vi "Read in last_sessionXML.vi"(8 "error in":errorcluster) -> (0 "error out":errorcluster, 3 "All Controlls For Saving":T1={"Confocal Controls"={"Channel Selection"=enum."A", "Pixel Count"={"Pixels in X"=512, "Pixels in Y"=512}, "Field Size"=174.0, "Frames"=0, "Averaging"=FALSE, "Alignment"=0.0, "Scan Mode"=TRUE, "Gain"={"Gain A"=0, "Gain B"=0}, "Enable PMTs"={"A"=TRUE, "B"=TRUE}, "Voltage Range"={"Range A"=10, "Range B"=10}, "Multi Frame Count"=0.0, "Trigger Mode"=2.0, "Real Time Averaging"=TRUE, "PFOV"=0.0, "MicronsPerPx"=0.0}, "iFlex Control"={"561"=0.0, "488"=0.0, "Global Shutter"=FALSE, "561 Shutter"=FALSE}, "PIFOC Settings"={"PIFOC Position (mm) [SET]"=0.0, "PIFOC Position\n(um) [ACT]"=0.0087, "last command"=""}, "PinSelector"=6.0, "Manlight Controls"={"Manlight Power"=0.0, "Open Serial"=FALSE, "VISA Refnum"=""}, "Exp Params"={"Experiment Type"="2D Snapshot", "Experiment Name"="Experiment_1", "ExpPath"=path "E:/Data", "TSFrames"=1000, "TSfps"=1000, "ZTSFrames"=1000, "ZTSdt"=1, "Streaming"=FALSE, "Z Stack Settings"={"Start"=0.0, "Step Size"=0.1, "Finish"=1.0}, "total images"=1, "tdms ref"=refnum, "frame #"=0, "images per stack"=1, "total stacks"=1, "period"=1, "PI MVR Increment"=""}, "Spots"=[]} {"Spots"."Z" format="%_4g"; "Spots"."Y" format="%_4g"; "Spots"."X" format="%_4g"; "Spots"."Phase" format="%_4g"; "Spots"."Intensity" format="%_4g"; "Exp Params"."period" min=1; "Exp Params"."total stacks" min=1; "Exp Params"."images per stack" min=1; "Exp Params"."total images" min=1; "Exp Params"."Z Stack Settings"."Start" min=0.0 max=100.0 step=0.1; "Exp Params"."Z Stack Settings"."Step Size" min=0.1 max=100.0 step=0.1; "Exp Params"."Z Stack Settings"."Finish" min=0.0 max=100.0 step=0.1; "Exp Params"."TSFrames" min=1 step=1; "Exp Params"."ZTSdt" min=1 step=1; "Exp Params"."ZTSFrames" min=2 step=1; "Exp Params"."TSfps" min=1 max=1000 step=1; "Manlight Controls"."Manlight Power" min=0.0 max=10.0 step=0.1 scale=0.0..10.0; "PinSelector" items=["25", "30", "35", "40", "45", "50", "60", "70", "80", "90", "100", "125", "200", "300", "1000", "2000"]; "PIFOC Settings"."PIFOC Position\n(um) [ACT]" format="%.2f"; "PIFOC Settings"."PIFOC Position (mm) [SET]" min=0.0 max=100.0 step=0.1 scale=0.0..100.0; "iFlex Control"."561" min=12.5 max=100.0 step=0.1 scale=0.0..100.0; "iFlex Control"."488" min=30.0 max=100.0 step=0.1 scale=0.0..100.0; "Confocal Controls"."Field Size" min=5.0 max=255.0 step=1.0 scale=5.0..255.0; "Confocal Controls"."PFOV" min=1.0 max=300.0 step=0.1; "Confocal Controls"."MicronsPerPx" min=0.01 step=0.01 format="%.2f"; "Confocal Controls"."Gain"."Gain B" min=1 max=100 step=1; "Confocal Controls"."Gain"."Gain A" min=1 max=100 step=1; "Confocal Controls"."Voltage Range"."Range B" items=["100mV"=5, "200mV"=6, "400mV"=7, "1V"=10, "2V"=11, "4V"=12]; "Confocal Controls"."Voltage Range"."Range A" items=["100mV"=5, "200mV"=6, "400mV"=7, "1V"=10, "2V"=11, "4V"=12]; "Confocal Controls"."Pixel Count"."Pixels in Y" items=["32"=32, "64"=64, "128"=128, "256"=256, "512"=512, "1024"=1024, "2048"=2048]; "Confocal Controls"."Pixel Count"."Pixels in X" items=["32"=32, "64"=64, "128"=128, "256"=256, "512"=512, "1024"=1024, "2048"=2048]})   [LabVIEW 2020]
uses:
  _Controls/All Controls For Saving.ctl
  _Controls/Confocal Controls.ctl
  _Controls/iFlex.ctl
  _Controls/PIFOC Position.ctl
  _Controls/Manlight Controls.ctl
  _Controls/Exp Params.ctl
  _Controls/Spots.ctl
  <vilib>/Utility/xml.llb/Read From XML File(string).vi
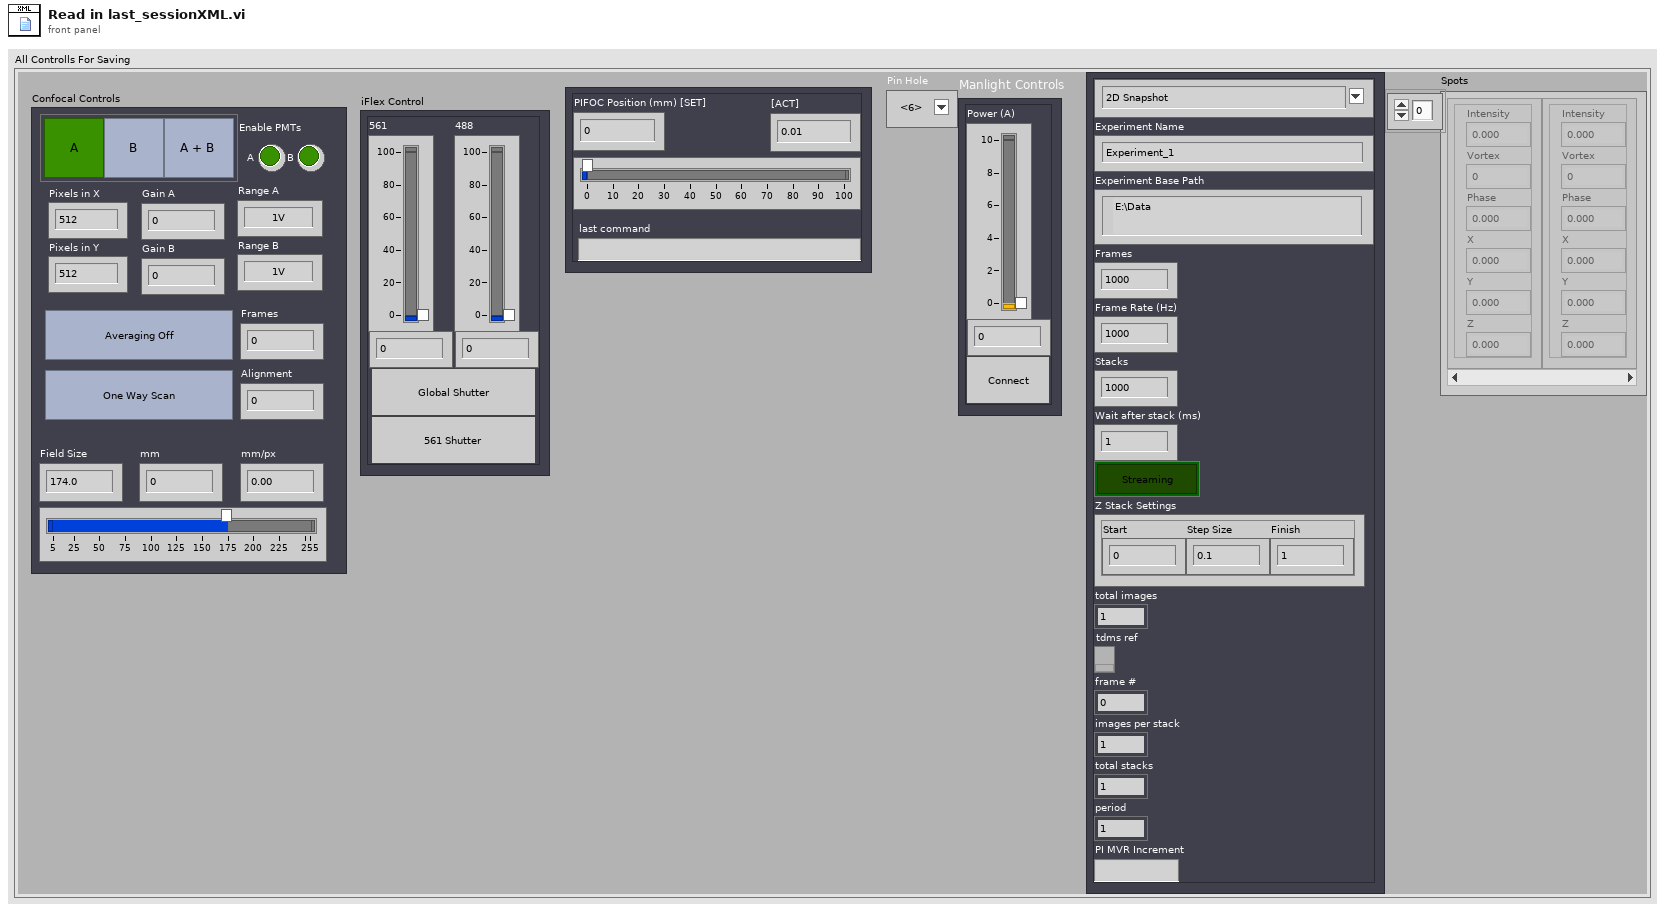
[diagram p1: front panel]
types:
  T1 = typedef "All Controls For Saving.ctl" = cluster{"Confocal Controls":T2, "iFlex Control":T3, "PIFOC Settings":T4, "PinSelector":dbl, "Manlight Controls":T5, "Exp Params":T6, "Spots":T7}
  T2 = typedef "Confocal Controls.ctl" = cluster{"Channel Selection":enum32{"A", "B", "AB"}, "Pixel Count":cluster{"Pixels in X":u32, "Pixels in Y":u32}, "Field Size":dbl, "Frames":u8, "Averaging":bool, "Alignment":dbl, "Scan Mode":bool, "Gain":cluster{"Gain A":u8, "Gain B":u8}, "Enable PMTs":cluster{"A":bool, "B":bool}, "Voltage Range":cluster{"Range A":u16, "Range B":u16}, "Multi Frame Count":dbl, "Trigger Mode":dbl, "Real Time Averaging":bool, "PFOV":dbl, "MicronsPerPx":dbl}
  T3 = typedef "iFlex.ctl" = cluster{"561":dbl, "488":dbl, "Global Shutter":bool, "561 Shutter":bool}
  T4 = typedef "PIFOC Position.ctl" = cluster{"PIFOC Position (mm) [SET]":dbl, "PIFOC Position\n(um) [ACT]":dbl, "last command":string}
  T5 = typedef "Manlight Controls.ctl" = cluster{"Manlight Power":dbl, "Open Serial":bool, "VISA Refnum":refnum<visa-resource-name>}
  T6 = typedef "Exp Params.ctl" = cluster{"Experiment Type":string, "Experiment Name":string, "ExpPath":path, "TSFrames":i32, "TSfps":i32, "ZTSFrames":i32, "ZTSdt":i32, "Streaming":bool, "Z Stack Settings":cluster{"Start":dbl, "Step Size":dbl, "Finish":dbl}, "total images":i32, "tdms ref":refnum<k34>, "frame #":i64, "images per stack":i32, "total stacks":i32, "period":i32, "PI MVR Increment":string}
  T7 = typedef "Spots.ctl" = cluster{"Intensity":dbl, "Vortex":dbl, "Phase":dbl, "X":dbl, "Y":dbl, "Z":dbl}[]
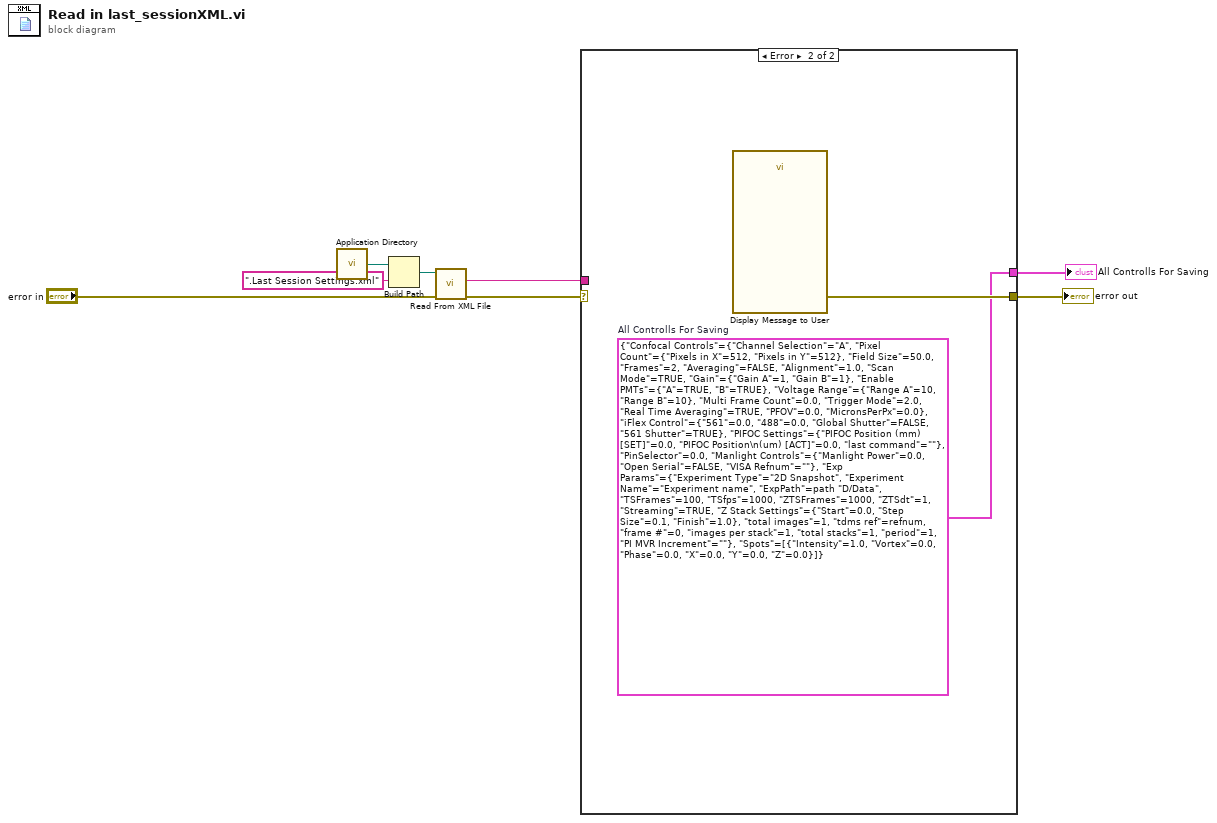
[diagram p0: block diagram]
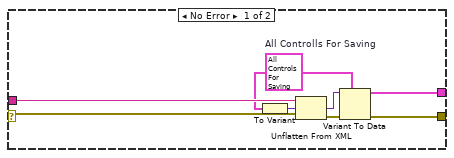
[diagram p2: hidden frame]
diagram:
  n1 = call <vilib>:"Application Directory.vi"() -> ("Application Directory"=w5:path)
  n2 = Build Path(base path=w5, name or relative path=".Last Session Settings.xml") -> (appended path=w7:path)
  n3 = call-poly <vilib>:"Read From XML File.vi"("error in (no error)"="error in", "XML File Path"=w7) -> ("error out"=w1:errorcluster, "XML Elements"=w2:string)  [unwired: 7 in, 1 out]
  n4 = case shown="Error" w1 {
    selector: w1 -> [w10 _]
    tunnel: [w16 w18] -> w4
    tunnel: [w15 w17] -> w3
    tunnel: w2 -> [w13 _]
    frame No Error {
      w12 = T1 {"Confocal Controls"={"Channel Selection"=enum."A", "Pixel Count"={"Pixels in X"=512, "Pixels in Y"=512}, "Field Size"=0.0, "Frames"=0, "Averaging"=FALSE, "Alignment"=0.0, "Scan Mode"=FALSE, "Gain"={"Gain A"=0, "Gain B"=0}, "Enable PMTs"={"A"=FALSE, "B"=FALSE}, "Voltage Range"={"Range A"=10, "Range B"=10}, "Multi Frame Count"=0.0, "Trigger Mode"=0.0, "Real Time Averaging"=FALSE, "PFOV"=0.0, "MicronsPerPx"=0.0}, "iFlex Control"={"561"=0.0, "488"=0.0, "Global Shutter"=FALSE, "561 Shutter"=FALSE}, "PIFOC Settings"={"PIFOC Position (mm) [SET]"=0.0, "PIFOC Position\n(um) [ACT]"=0.0087, "last command"=""}, "PinSelector"=6.0, "Manlight Controls"={"Manlight Power"=0.0, "Open Serial"=FALSE, "VISA Refnum"=""}, "Exp Params"={"Experiment Type"="2D Snapshot", "Experiment Name"="Experiment_1", "ExpPath"=path "E:/Data", "TSFrames"=1000, "TSfps"=1000, "ZTSFrames"=1000, "ZTSdt"=1, "Streaming"=FALSE, "Z Stack Settings"={"Start"=0.0, "Step Size"=0.1, "Finish"=1.0}, "total images"=1, "tdms ref"=refnum, "frame #"=0, "images per stack"=1, "total stacks"=1, "period"=1, "PI MVR Increment"=""}, "Spots"=[]}  # All Controlls For Saving
      n5 = To Variant(anything=w12) -> (Variant=w14:variant)
      n6 = Unflatten From XML(xml string=w13, type=w14, error in (no error)=w10) -> (value=w11:variant, error out=w9:errorcluster)
      n7 = Variant To Data(error in=w9, type=w12, Variant=w11) -> (data=w15:T1, error out=w16:errorcluster)
    }
    frame Error {
      w17 = T1 {"Confocal Controls"={"Channel Selection"=enum."A", "Pixel Count"={"Pixels in X"=512, "Pixels in Y"=512}, "Field Size"=50.0, "Frames"=2, "Averaging"=FALSE, "Alignment"=1.0, "Scan Mode"=TRUE, "Gain"={"Gain A"=1, "Gain B"=1}, "Enable PMTs"={"A"=TRUE, "B"=TRUE}, "Voltage Range"={"Range A"=10, "Range B"=10}, "Multi Frame Count"=0.0, "Trigger Mode"=2.0, "Real Time Averaging"=TRUE, "PFOV"=0.0, "MicronsPerPx"=0.0}, "iFlex Control"={"561"=0.0, "488"=0.0, "Global Shutter"=FALSE, "561 Shutter"=TRUE}, "PIFOC Settings"={"PIFOC Position (mm) [SET]"=0.0, "PIFOC Position\n(um) [ACT]"=0.0, "last command"=""}, "PinSelector"=0.0, "Manlight Controls"={"Manlight Power"=0.0, "Open Serial"=FALSE, "VISA Refnum"=""}, "Exp Params"={"Experiment Type"="2D Snapshot", "Experiment Name"="Experiment name", "ExpPath"=path "D:/Data", "TSFrames"=100, "TSfps"=1000, "ZTSFrames"=1000, "ZTSdt"=1, "Streaming"=TRUE, "Z Stack Settings"={"Start"=0.0, "Step Size"=0.1, "Finish"=1.0}, "total images"=1, "tdms ref"=refnum, "frame #"=0, "images per stack"=1, "total stacks"=1, "period"=1, "PI MVR Increment"=""}, "Spots"=[{"Intensity"=1.0, "Vortex"=0.0, "Phase"=0.0, "X"=0.0, "Y"=0.0, "Z"=0.0}]}  # All Controlls For Saving
      n8 = call "Display Message to User"() -> ("error out"=w18:errorcluster)  [unwired: 10 in, 1 out]
    }
  }
  "error out" <- w4
  "All Controlls For Saving" <- w3
